vi "STED Control V7.vi"(7 "Calling VI Ref":refnum<vi>) -> ()   [LabVIEW 2016]
uses:
  FPGA-7842R-Reference.ctl
  Scan Parameters.ctl
  Manual Controls V2.ctl
  Laser Controls.ctl
  <vilib>/vision/Image Controls.llb/IMAQ Image.ctl
  <vilib>/Utility/miscctls.llb/LVPointTypeDef.ctl
  Type Defs/Image Acquisition Parameters.ctl
  Detectors.ctl
  Focus Control.ctl
panel:
  in  "File Name":string
  in  "Focus Control":T1
  in  "Detectors":T2
  in  "Laser Controls":T3 {"405 Power (0-5V)" min=0.0 max=5.0}
  in  "Save Path":path
  in  "Capture":bool
  in  "Image Acquisition Parameters":T4={"Scan Type"=enum."Beam Scanning", "Scan Mode"=enum."XY", "Fast Axis Frequency (Hz)"=16110.0, "Image Format"=256, "Line Accumulations"=100, "Frames Per Capture"=1, "Frames Accumulations"=1, "Image Dimension (um)"=[15.0, 15.0], "Number of Z Steps"=1, "Z Steps Size (um)"=1.0, "Pixel Size (nm)"=[58.59375, 58.59375]} {"Z Steps Size (um)" min=0.0; "Number of Z Steps" min=1; "Frames Accumulations" min=1; "Frames Per Capture" min=1; "Line Accumulations" min=1; "Image Format" items=["64 x 64"=64, "128 x 128"=128, "256 x 256"=256, "512 x 512"=512, "1024 x 1024"=1024, "2048 x 2048"=2048]}
  in  "Live":bool
  in  "Quit":bool
  # "Copyright (C) 2020 Edward S Allgeyer\n\nRedistribution and use in source and binary forms, with or without\nmodification, are permitted provided that the following conditions\nare met:\n\n1. Redistributions of source code must retain the above copyright\n   notice, this list of conditions and the following disclaimer.\n\n2. Redistributions in binary form must reproduce the above copyright\n   notice, this list of conditions and the following disclaimer in\n   the documentation and/or other materials provided with the\n   distribution.\n\n3. Neither the name of the copyright holder nor the names of its\n   contributors may be used to endorse or promote products derived\n   from this software without specific prior written permission.\n\nTHIS SOFTWARE IS PROVIDED BY THE COPYRIGHT HOLDERS AND CONTRIBUTORS\n\"AS IS\" AND ANY EXPRESS OR IMPLIED WARRANTIES, INCLUDING, BUT NOT\nLIMITED TO, THE IMPLIED WARRANTIES OF MERCHANTABILITY AND FITNESS\nFOR A PARTICULAR PURPOSE ARE DISCLAIMED. IN NO EVENT SHALL THE\nCOPYRIGHT HOLDER OR CONTRIBUTORS BE LIABLE FOR ANY DIRECT, INDIRECT,\nINCIDENTAL, SPECIAL, EXEMPLARY, OR CONSEQUENTIAL DAMAGES (INCLUDING,\nBUT NOT LIMITED TO, PROCUREMENT OF SUBSTITUTE GOODS OR SERVICES;\nLOSS OF USE, DATA, OR PROFITS; OR BUSINESS INTERRUPTION) HOWEVER\nCAUSED AND ON ANY THEORY OF LIABILITY, WHETHER IN CONTRACT, STRICT\nLIABILITY, OR TORT (INCLUDING NEGLIGENCE OR OTHERWISE) ARISING IN\nANY WAY OUT OF THE USE OF THIS SOFTWARE, EVEN IF ADVISED OF THE\nPOSSIBILITY OF SUCH DAMAGE."
  # "XY"
  # "Z"
  # "Length"
  # "Height"
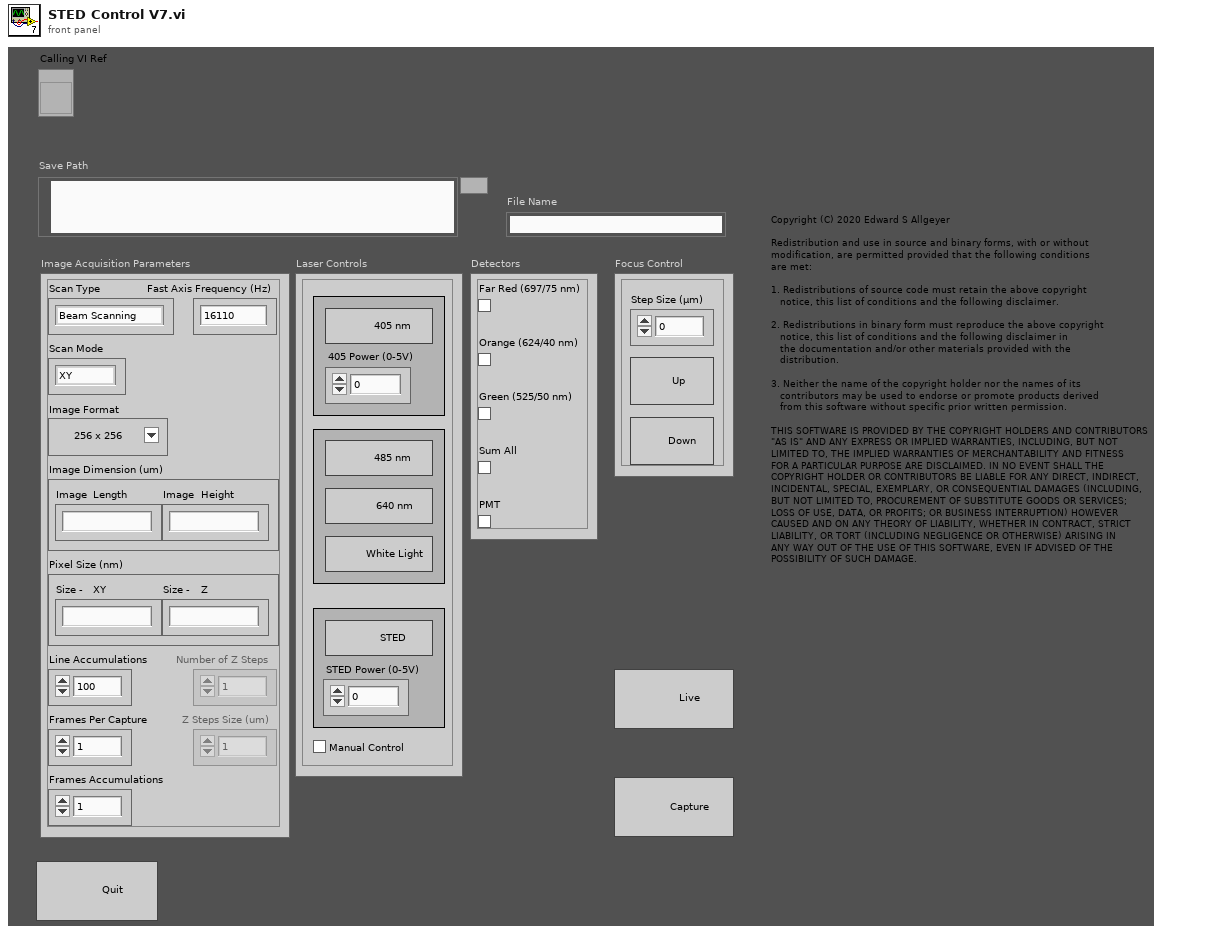
[diagram p1: front panel]
types:
  T1 = typedef "Focus Control.ctl" = cluster{"ZoomUp":bool, "ZoomDown":bool, "SetZoom":bool, "Step Size (µm)":dbl}
  T2 = typedef "Detectors.ctl" = cluster{"PMT":bool, "Far Red (697/75 nm)":bool, "Orange (624/40 nm)":bool, "Green (525/50 nm)":bool, "Sum All":bool}
  T3 = typedef "Laser Controls.ctl" = cluster{"STED Power (0-5V)":dbl, "STED":bool, "640 nm":bool, "485 nm":bool, "Manual Control":bool, "White Light":bool, "405 nm":bool, "405 Power (0-5V)":dbl}
  T4 = typedef "Image Acquisition Parameters.ctl" = cluster{"Scan Type":enum16{"Sample Scanning", "Beam Scanning"}, "Scan Mode":enum16{"XY", "XZ", "YZ", "XYZ"}, "Fast Axis Frequency (Hz)":dbl, "Image Format":u16, "Line Accumulations":u16, "Frames Per Capture":u16, "Frames Accumulations":u16, "Image Dimension (um)":dbl[], "Number of Z Steps":u8, "Z Steps Size (um)":dbl, "Pixel Size (nm)":dbl[]}
  T5 = enum8{"Enabled", "Disabled", "Disabled and Grayed Out"}
  T6 = enum16{"Always On", "Always Off", "Off While Running"}
  T7 = typedef "LVPointTypeDef.ctl" = cluster{"Horizontal":i16, "Vertical":i16}
  T8 = typedef "Manual Controls V2.ctl" = cluster{"Galvo 1 Position (I16)":i16, "Galvo 2 Position (I16)":i16, "X Axis Voltage (I16)":i16, "Y Axis Voltage (I16)":i16, "Z Axis Voltage (I16)":i16, "Res Mirror Amp (I16)":i16, "Res Mirror Mute":bool}
  T9 = typedef "Scan Parameters.ctl" = cluster{"Fast_Ax_Amp_V":dbl, "Fast_Ax_Off_V":dbl, "Slow_Ax_Amp_V":dbl, "Slow_Ax_Off_V ":dbl, "Slow_Ax_Max_V_VperS":dbl, "Slow_Ax1_Del25ns":i32, "Slow_Ax2_Del25ns":i32, "Stage_X_Off_V":dbl, "Stage_Y_Off_V":dbl, "Stage_Z_Off_V":dbl, "Galvo1_Off_V":dbl, "Galvo2_Off_V":dbl, "Last_Scan_Mode":enum16{"XY", "XZ", "YZ", "XYZ"}, "Current_Scan_Mode":enum16{"XY", "XZ", "YZ", "XYZ"}, "Fly_Back_Lines":u16, "Linear_Ramp_End":u32, "Z_Step_I16":i16, "Z_Start_I16":i16, "Laser_States _U32":u32, "590_Voltage_I16":i16, "775_AOM_Volt_I16":i16, "Blanking OFF":bool, "Unused_Axis_I16":i16}
  T10 = typedef "FPGA-7842R-Reference.ctl" = enum16{"Stage Control", "Laser Control", "Unused Axis I16", "Exit", "Set Res Mirror", "Set Galvo", "Default", "Close FPGA", "Stop Waveforms", "Start Waveforms", "Initialize"}
  T11 = typedef "LVRectTypeDef.ctl" = cluster{"Left":i16, "Top":i16, "Right":i16, "Bottom":i16}
  T12 = typedef "LVBoundsTypeDef.ctl" = cluster{"Width":u32, "Height":u32}
  T13 = cluster{"Scan Type":bool, "Scan Mode":bool, "Fast Axis Frequency (Hz)":bool, "Image Format":bool, "Line Accumulations":bool, "Frames Per Capture":bool, "Frames Accumulations":bool, "Image Dimension (um)":bool[], "Number of Z Steps":bool, "Z Steps Size (um)":bool, "Pixel Size (nm)":bool[]}
  T14 = typedef "Scanning Conversions.ctl" = cluster{"Stage X Axis (Volts/um)":dbl, "Stage Y Axis (Volts/um)":dbl, "Stage Z Axis (Volts/um)":dbl}
  T15 = typedef "IMAQ Image.ctl" = refnum<image>
  T16 = typedef "Waveform Data.ctl" = cluster{"Waveform Scan Parameters":cluster{"Scanning Mode":u8, "Fast Axis WF Length (Elements)":i32, "Fast Axis Sample Period (Ticks)":u32, "Slow Axis 1 WF Length (Elements)":i32, "Slow Axis 1 Sample Period (Ticks)":u32, "Slow Axis 1 Delay (25 ns) Steps":i32, "Slow Axis 2 WFLength (Elements)":i32, "Slow Axis 2 Sample Period (Ticks)":u32, "Slow Axis 2 Delay (25 ns) Steps":i32}, "Fast Axis Waveform":dbl[], "Slow Axis 1 Waveform":dbl[], "Slow Axis 2 Waveform":dbl[]}
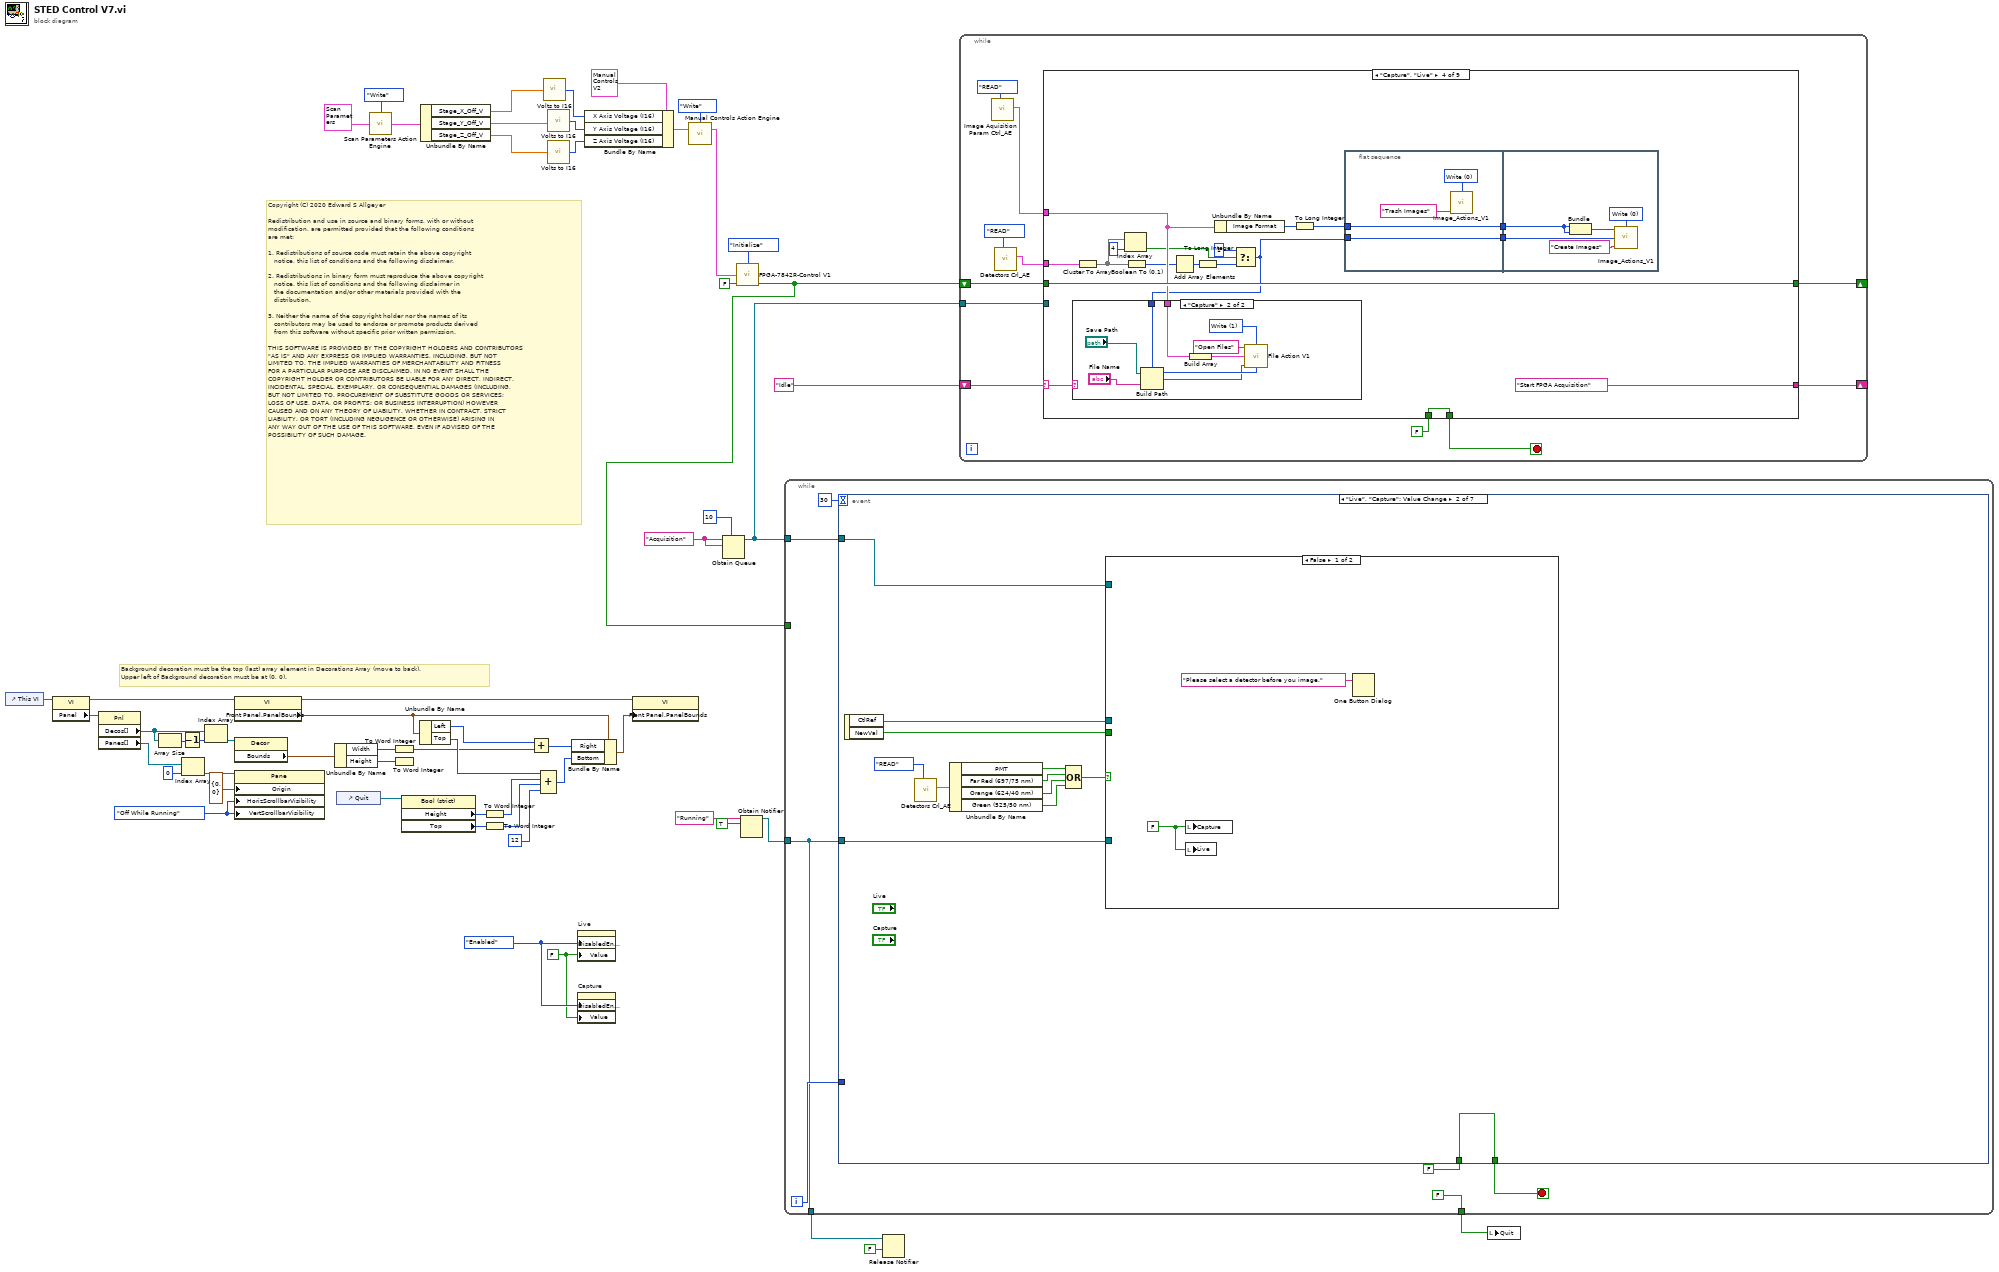
[diagram p0: block diagram]
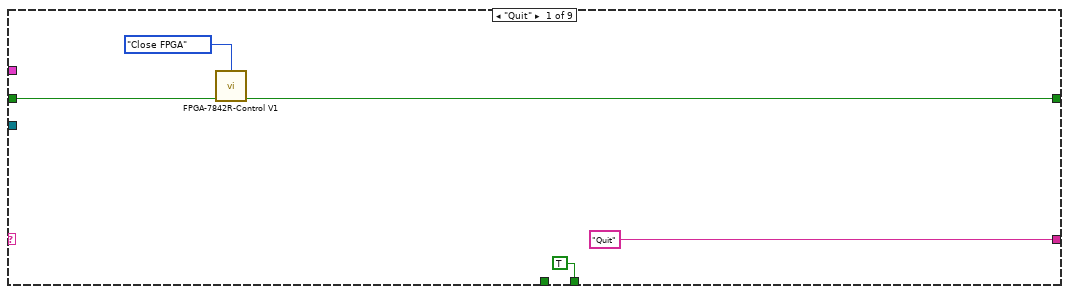
[diagram p2: hidden frame]
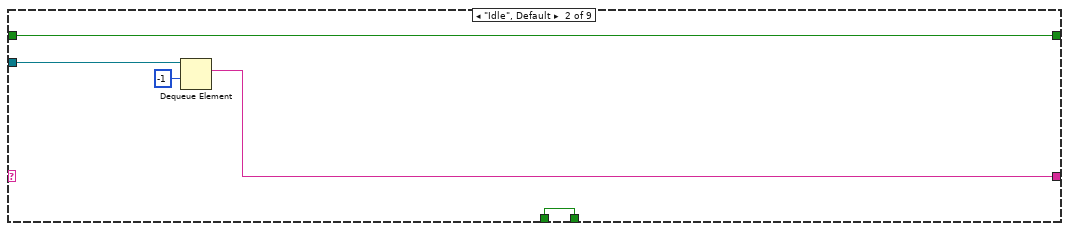
[diagram p3: hidden frame]
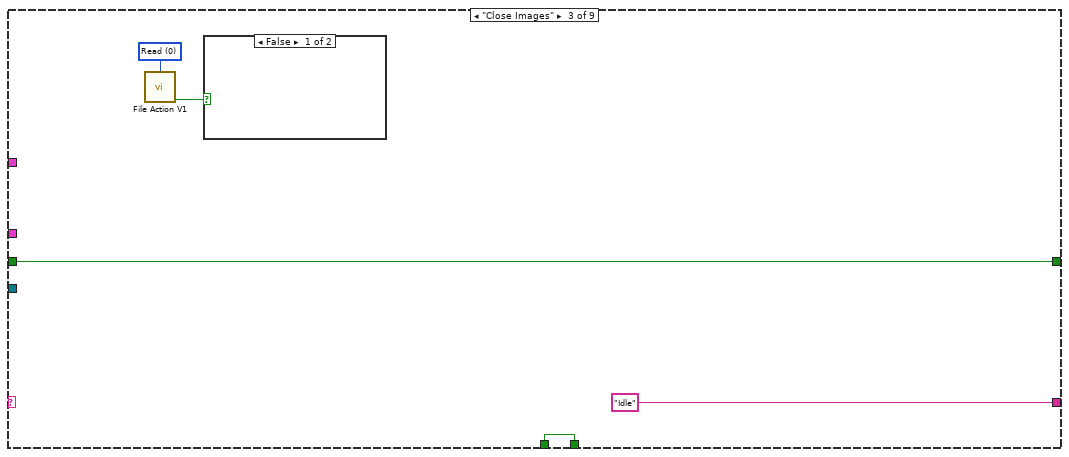
[diagram p4: hidden frame]
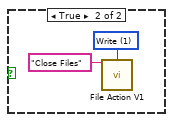
[diagram p5: hidden frame]
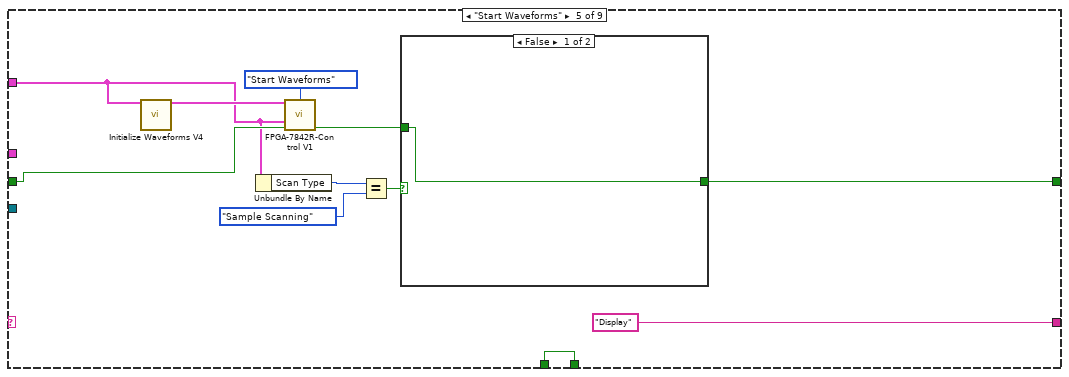
[diagram p7: hidden frame]
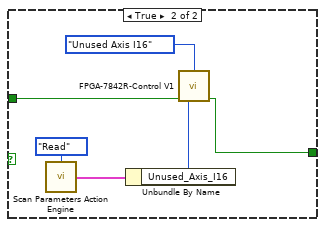
[diagram p8: hidden frame]
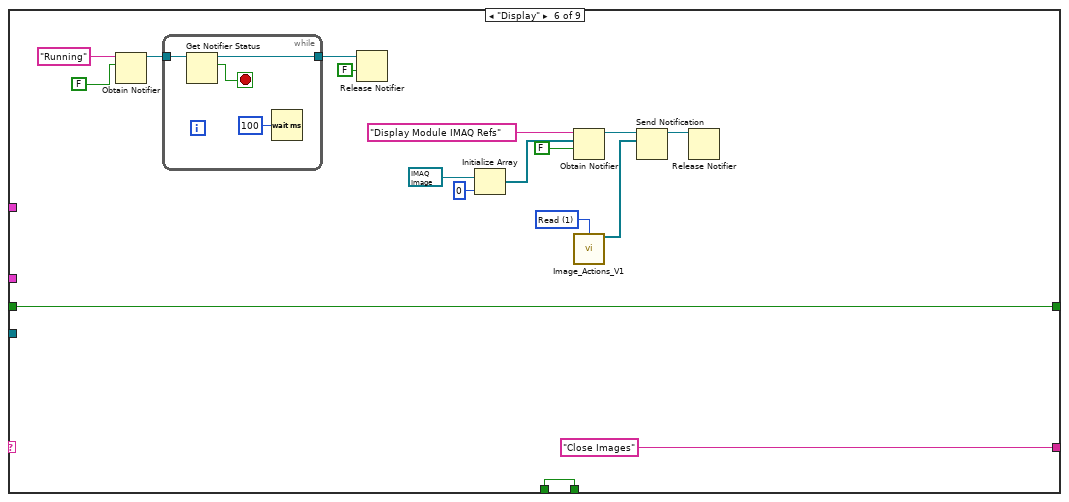
[diagram p9: hidden frame]
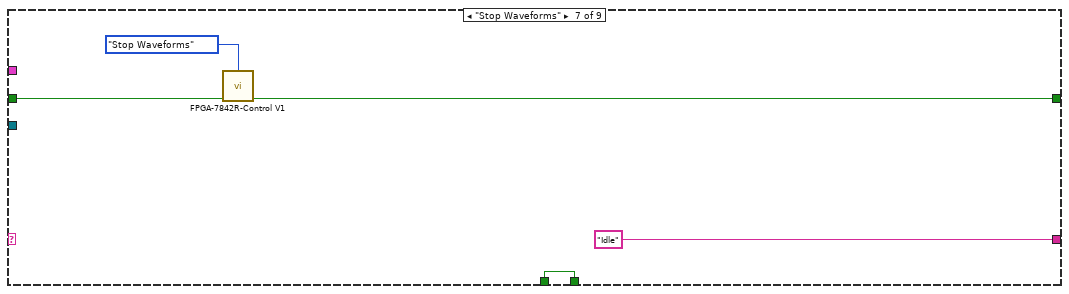
[diagram p10: hidden frame]
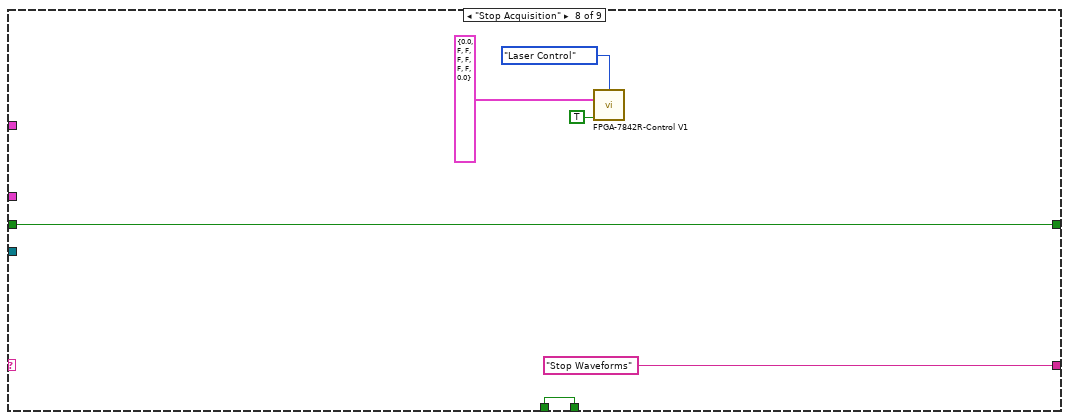
[diagram p11: hidden frame]
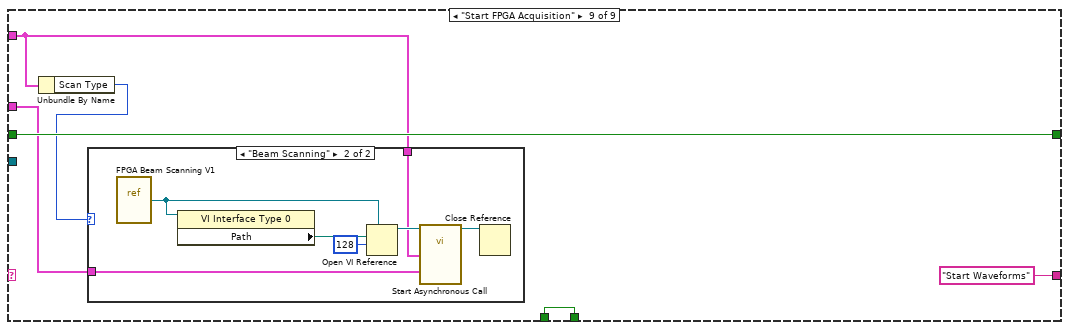
[diagram p12: hidden frame]
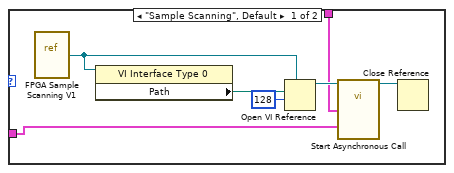
[diagram p13: hidden frame]
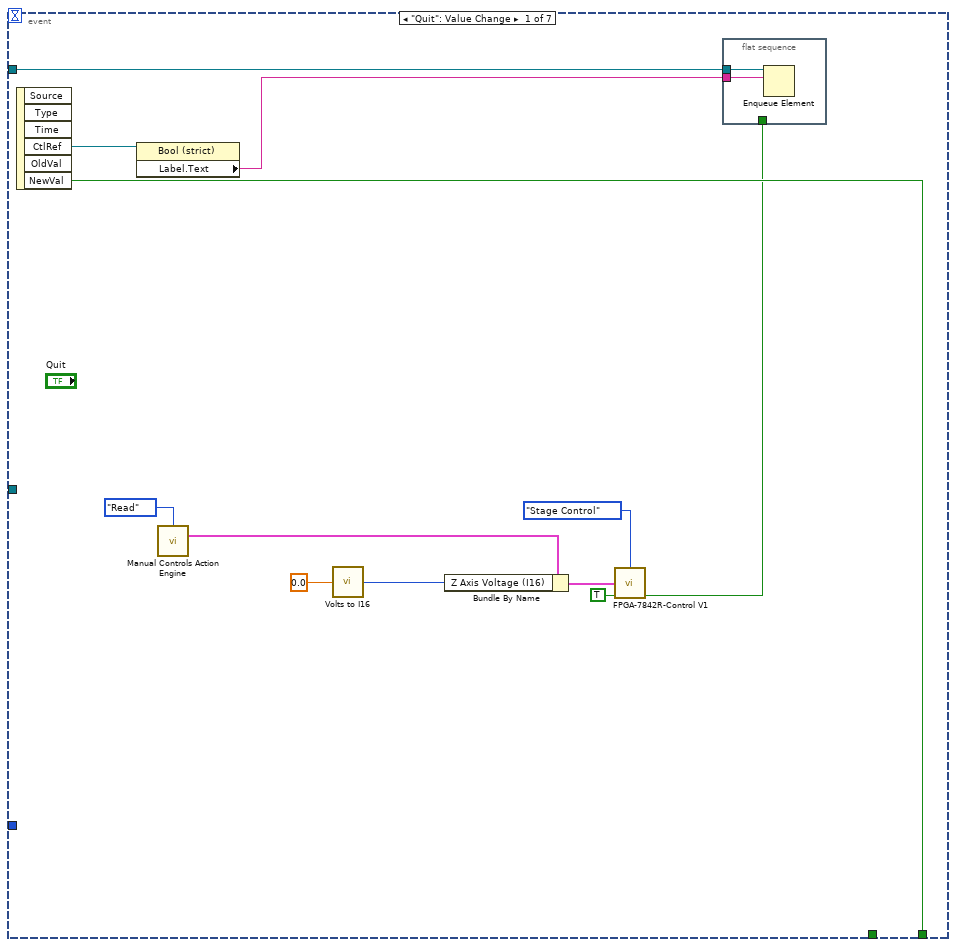
[diagram p14: hidden frame]
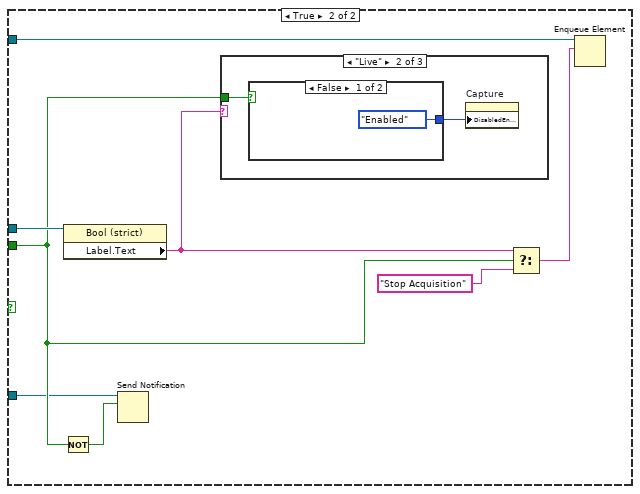
[diagram p15: hidden frame]
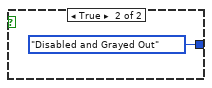
[diagram p17: hidden frame]
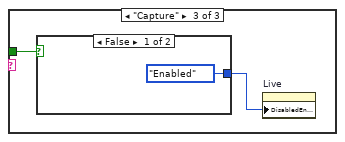
[diagram p18: hidden frame]
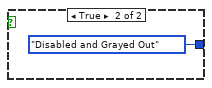
[diagram p19: hidden frame]
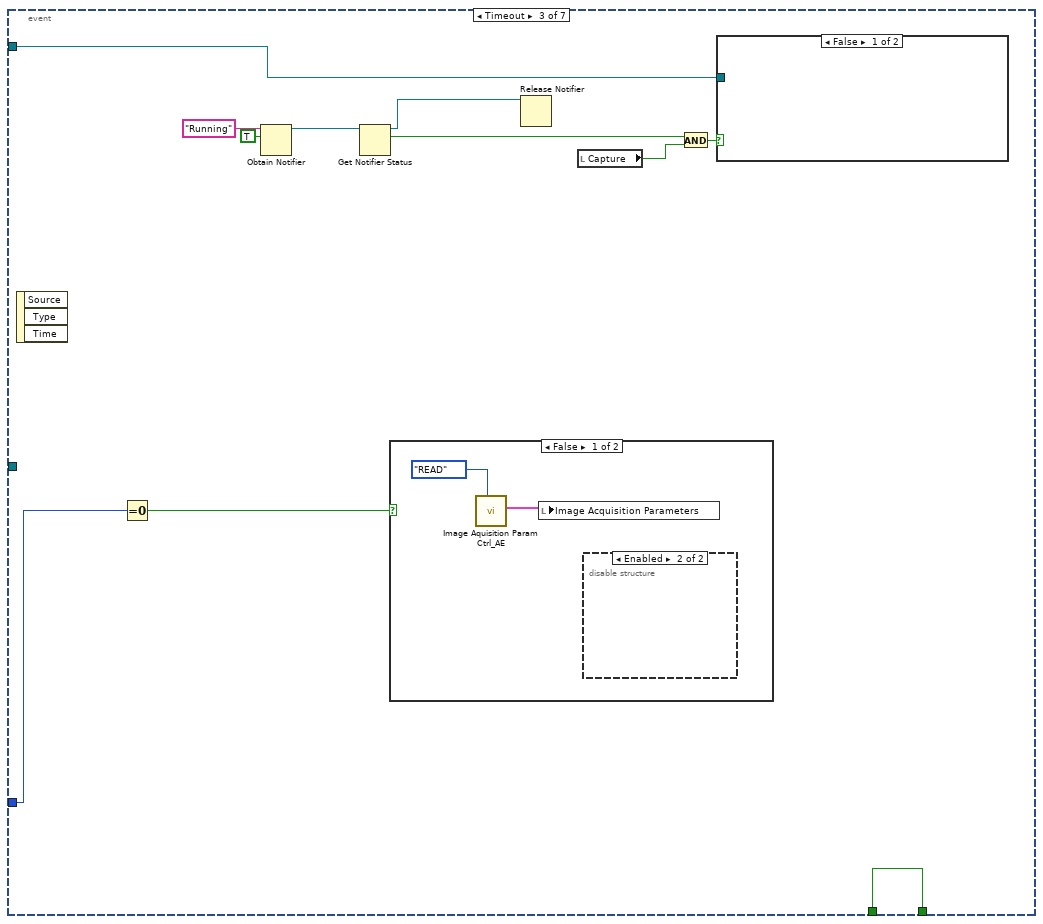
[diagram p20: hidden frame]
diagram:
  w1 = FALSE ("Live")
  w2 = T5."Enabled" ("Disabled")
  w15 = T6."Off While Running" ("Vertical Scrollbar Visibility")
  w56 = "Acquisition" ("name (unnamed)")
  # "Copyright (C) 2020 Edward S Allgeyer\n\nRedistribution and use in source and binary forms, with or without\nmodification, are permitted provided that the following conditions\nare met:\n\n1. Redistributions of source code must retain the above copyright\n   notice, this list of conditions and the following disclaimer.\n\n2. Redistributions in binary form must reproduce the above copyright\n   notice, this list of conditions and the following disclaimer in\n   the documentation and/or other materials provided with the\n   distribution.\n\n3. Neither the name of the copyright holder nor the names of its\n   contributors may be used to endorse or promote products derived\n   from this software without specific prior written permission.\n\nTHIS SOFTWARE IS PROVIDED BY THE COPYRIGHT HOLDERS AND CONTRIBUTORS\n\"AS IS\" AND ANY EXPRESS OR IMPLIED WARRANTIES, INCLUDING, BUT NOT\nLIMITED TO, THE IMPLIED WARRANTIES OF MERCHANTABILITY AND FITNESS\nFOR A PARTICULAR PURPOSE ARE DISCLAIMED. IN NO EVENT SHALL THE\nCOPYRIGHT HOLDER OR CONTRIBUTORS BE LIABLE FOR ANY DIRECT, INDIRECT,\nINCIDENTAL, SPECIAL, EXEMPLARY, OR CONSEQUENTIAL DAMAGES (INCLUDING,\nBUT NOT LIMITED TO, PROCUREMENT OF SUBSTITUTE GOODS OR SERVICES;\nLOSS OF USE, DATA, OR PROFITS; OR BUSINESS INTERRUPTION) HOWEVER\nCAUSED AND ON ANY THEORY OF LIABILITY, WHETHER IN CONTRACT, STRICT\nLIABILITY, OR TORT (INCLUDING NEGLIGENCE OR OTHERWISE) ARISING IN\nANY WAY OUT OF THE USE OF THIS SOFTWARE, EVEN IF ADVISED OF THE\nPOSSIBILITY OF SUCH DAMAGE."
  # "Background decoration must be the top (last) array element in Decorations Array (move to back).\nUpper left of Background decoration must be at (0, 0)."
  n1 = control-ref of="This VI"() -> (w7:refnum<vi>)
  n2 = property class="VI"(reference=w7) -> (reference out=w16:refnum<vi>, "Panel"=w8:refnum<vi>)  [unwired: 1 in, 1 out]
  n3 = property class="Pnl"(reference=w8) -> ("Decos[]"=w6:refnum<vi>[], "Panes[]"=w12:refnum<vi>[])  [unwired: 1 in, 2 out]
  n4 = Array Size(array=w6) -> (size(s)=w4:i32)
  n5 = Decrement(x=w4) -> (x-1=w5:i32)
  n6 = Index Array(array=w12, index=0) -> (element=w11:refnum<vi>)
  n7 = Index Array(array=w6, index=w5) -> (element=w14:refnum<vi>)
  n8 = property class="VI"(reference=w16) -> (reference out=w18:refnum<vi>, "Front Panel.PanelBounds"=w19:T11)  [unwired: 1 in, 1 out]
  n9 = property class="Decor"(reference=w14) -> ("Bounds"=w17:T12)  [unwired: 1 in, 2 out]
  n10 = property class="Pane"(reference=w11, "Origin"=T7 {"Horizontal"=0, "Vertical"=0}, "HorizScrollbarVisibility"=w15, "VertScrollbarVisibility"=w15) -> ()  [unwired: 1 in, 2 out]
  n11 = Unbundle By Name(w17) -> ("Width"=w22:u32, "Height"=w25:u32)
  n12 = control-ref of="Quit"() -> (w9:refnum<vi>)
  n13 = call "Scan Parameters Action Engine.vi"("Action"=enum16{"Read", "Write"}."Write", "Scan Parameters IN"=T9 {"Fast_Ax_Amp_V"=0.0, "Fast_Ax_Off_V"=0.0, "Slow_Ax_Amp_V"=0.0, "Slow_Ax_Off_V "=0.0, "Slow_Ax_Max_V_VperS"=0.0, "Slow_Ax1_Del25ns"=0, "Slow_Ax2_Del25ns"=0, "Stage_X_Off_V"=5.0, "Stage_Y_Off_V"=5.0, "Stage_Z_Off_V"=5.0, "Galvo1_Off_V"=0.0, "Galvo2_Off_V"=0.0, "Last_Scan_Mode"=enum."XY", "Current_Scan_Mode"=enum."XY", "Fly_Back_Lines"=0, "Linear_Ramp_End"=0, "Z_Step_I16"=0, "Z_Start_I16"=0, "Laser_States _U32"=0, "590_Voltage_I16"=0, "775_AOM_Volt_I16"=0, "Blanking OFF"=FALSE, "Unused_Axis_I16"=16384}) -> ("Scan Parameters OUT"=w45:T9)  [unwired: 13 in]
  n14 = To Word Integer(number=w22) -> (16bit integer=w24:i16)
  n15 = To Word Integer(number=w25) -> ()  [unwired: 1 out]
  n16 = property class="Bool (strict)"(reference=w9) -> ("Height"=w27:u32, "Top"=w28:i32)  [unwired: 1 in, 2 out]
  n17 = Unbundle By Name(w19) -> ("Left"=w21:i16, "Top"=w32:i16)
  n18 = Unbundle By Name(w45) -> ("Stage_X_Off_V"=w41:dbl, "Stage_Y_Off_V"=w40:dbl, "Stage_Z_Off_V"=w39:dbl)
  n19 = To Word Integer(number=w27) -> (16bit integer=w30:i16)
  n20 = To Word Integer(number=w28) -> (16bit integer=w31:i16)
  n21 = Add(x=w21, y=w24) -> (x+y=w23:i16)
  n22 = Compound Arithmetic op=ADD(w32, w30, w31, i16 12 ("y")) -> (w26:i16)
  n23 = call "Volts to I16.vi"("Voltage (V)"=w41) -> ("I16"=w42:i16)  [unwired: 13 in, 1 out]
  n24 = call "Volts to I16.vi"("Voltage (V)"=w40) -> ("I16"=w43:i16)  [unwired: 13 in, 1 out]
  n25 = call "Volts to I16.vi"("Voltage (V)"=w39) -> ("I16"=w44:i16)  [unwired: 13 in, 1 out]
  n26 = Bundle By Name(cluster=w19, "Right"=w23, "Bottom"=w26) -> (w20:T11)
  n27 = property on="Live" class="Bool (strict)"("DisabledEnum"=w2, "Value"=w1) -> ()  [unwired: 2 in, 2 out]
  n28 = property on="Capture" class="Bool (strict)"("DisabledEnum"=w2, "Value"=w1) -> ()  [unwired: 2 in, 2 out]
  n29 = Bundle By Name(cluster=T8 {"Galvo 1 Position (I16)"=-280, "Galvo 2 Position (I16)"=0, "X Axis Voltage (I16)"=16384, "Y Axis Voltage (I16)"=16384, "Z Axis Voltage (I16)"=16384, "Res Mirror Amp (I16)"=0, "Res Mirror Mute"=FALSE} ("Manual Controls"), "X Axis Voltage (I16)"=w42, "Y Axis Voltage (I16)"=w43, "Z Axis Voltage (I16)"=w44) -> (w46:T8)
  n30 = property class="VI"(reference=w18, "Front Panel.PanelBounds"=w20) -> ()  [unwired: 1 in, 2 out]
  n31 = call "Manual Controls Action Engine.vi"("Action"=enum16{"Read", "Write"}."Write", "Manual Controls In"=w46) -> ("Manual Controls Out"=w48:T8)  [unwired: 13 in]
  n32 = Obtain Queue(max queue size (-1, unlimited)=10, name (unnamed)=w56, element data type=w56) -> (queue out=w54:refnum<queue>)  [unwired: 2 in, 2 out]
  n33 = call "FPGA-7842R-Control V1.vi"("Action"=FPGA-7842R-Reference."Initialize", "Manual Controls"=w48, "Initialize"=FALSE) -> ("Initalized"=w33:bool)  [unwired: 12 in]
  n34 = Obtain Notifier(name (unnamed)="Running", notification data type=TRUE) -> (notifier out=w36:refnum<notifier>)  [unwired: 2 in, 2 out]
  n35 = while {
    tunnel: w54 -> [w62]
    tunnel: w36 -> [w59]
    tunnel: [w59] -> w34
    tunnel: w33 -> [_]
    tunnel: [FALSE] -> w3
    i -> [w60]
    stop <- w64 stop-if-true
    n36 = event shown="[1] \"Live\", \"Capture\": Value Change" {
      selector: _ -> [_ _ _ _ _ _ _]
      dyn-events: _ -> [_ _ _ _ _ _ _]
      timeout: 30 -> [_ _ _ _ _ _ _]
      tunnel: [w76 w90 w119 w138 w163 w199 w235] -> w64
      tunnel: FALSE -> [_ w90 w119 w138 w163 w199 w235]
      tunnel: w62 -> [w75 w89 w113 _ _ _ _]
      tunnel: w60 -> [_ _ w111 _ _ _ _]
      tunnel: w59 -> [_ w86 _ _ _ _ _]
      event "Quit": Value Change {
        n37 = event-data() -> ("CtlRef"=w74:refnum<vi>, "NewVal"=w76:bool)  [unwired: 1 in, 4 out]
        n38 = property class="Bool (strict)"(reference=w74) -> ("Label.Text"=w73:string)  [unwired: 1 in, 2 out]
        n39 = call "Manual Controls Action Engine.vi"("Action"=enum16{"Read", "Write"}."Read") -> ("Manual Controls Out"=w72:T8)  [unwired: 14 in]
        n40 = call "Volts to I16.vi"("Voltage (V)"=0.0) -> ("I16"=w65:i16)  [unwired: 13 in, 1 out]
        n41 = Bundle By Name(cluster=w72, "Z Axis Voltage (I16)"=w65) -> (w70:T8)
        n42 = call "FPGA-7842R-Control V1.vi"("Action"=FPGA-7842R-Reference."Stage Control", "Manual Controls"=w70, "Initialize"=TRUE) -> ("Initalized"=w66:bool)  [unwired: 12 in]
        n43 = flat-sequence {
          tunnel: w75 -> [w78]
          tunnel: w73 -> [w77]
          tunnel: w66 -> [_]
          frame #0 {
            n44 = Enqueue Element(queue=w78, element=w77) -> ()  [unwired: 2 in, 3 out]
          }
        }
      }
      event "Live", "Capture": Value Change {
        n45 = event-data() -> ("CtlRef"=w88:refnum<vi>, "NewVal"=w87:bool)  [unwired: 1 in]
        n46 = call "Detectors Crl_AE.vi"("Action"=enum16{"READ", "WRITE"}."READ") -> ("Detectors Parameters Out"=w84:T2)  [unwired: 10 in]
        n47 = Unbundle By Name(w84) -> ("PMT"=w83:bool, "Far Red (697/75 nm)"=w82:bool, "Orange (624/40 nm)"=w81:bool, "Green (525/50 nm)"=w80:bool)
        n48 = Compound Arithmetic op=OR(w83, w82, w81, w80) -> (w79:bool)
        n49 = case shown="False" w79 {
          tunnel: w89 -> [_ w100]
          tunnel: w88 -> [_ w99]
          tunnel: w87 -> [_ w94]
          tunnel: w86 -> [_ w93]
          frame False {
            w92 = FALSE ("Capture")
            n50 = local write "Capture"(w92) -> ()
            n51 = local write "Live"(w92) -> ()
            n52 = One Button Dialog(message="Please select a detector before you image.") -> ()  [unwired: 1 in, 1 out]
          }
          frame True {
            n53 = Not(x=w94) -> (.not. x?=w97:bool)
            n54 = property class="Bool (strict)"(reference=w99) -> ("Label.Text"=w95:string)  [unwired: 1 in, 2 out]
            n55 = Send Notification(notification=w97, notifier=w93) -> ()  [unwired: 1 in, 2 out]
            n56 = case shown="\"Live\"" w95 {
              tunnel: w94 -> [_ w101 w106]
              frame "False", Default {
              }
              frame "Live" {
                n57 = case shown="False" w101 {
                  tunnel: [T5."Enabled" ("Disabled") T5."Disabled and Grayed Out" ("Disabled")] -> w102
                  frame False {
                  }
                  frame True {
                  }
                }
                n58 = property on="Capture" class="Bool (strict)"("DisabledEnum"=w102) -> ()  [unwired: 2 in, 2 out]
              }
              frame "Capture" {
                n59 = case shown="False" w106 {
                  tunnel: [T5."Enabled" ("Disabled") T5."Disabled and Grayed Out" ("Disabled")] -> w105
                  frame False {
                  }
                  frame True {
                  }
                }
                n60 = property on="Live" class="Bool (strict)"("DisabledEnum"=w105) -> ()  [unwired: 2 in, 2 out]
              }
            }
            n61 = Select(t=w95, s=w94, f="Stop Acquisition") -> (s? t:f=w96:string)
            n62 = Enqueue Element(queue=w100, element=w96) -> ()  [unwired: 2 in, 3 out]
          }
        }
      }
      event Timeout {
        n63 = event-data() -> ()  [unwired: 1 in, 3 out]
        n64 = Equal To 0?(x=w111) -> (x = 0?=w110:bool)
        n65 = Obtain Notifier(name (unnamed)="Running", notification data type=TRUE) -> (notifier out=w117:refnum<notifier>)  [unwired: 2 in, 2 out]
        n66 = Get Notifier Status(notifier=w117) -> (notifier out=w109:refnum<notifier>, current notification=w115:bool)  [unwired: 1 in, 3 out]
        n67 = case shown="False" w110 {
          frame False {
            n68 = call "Image Aquisition Param Ctrl_AE.vi"("Action"=enum16{"READ", "WRITE"}."READ") -> ("Image Acquisition Parameters Out"=w121:T4)  [unwired: 10 in]
            n69 = local write "Image Acquisition Parameters"(w121) -> ()
            n70 = disable-structure shown="Enabled" {
              frame Disabled {
                n71 = call "FPGA-7842R-Control V1.vi"("Action"=FPGA-7842R-Reference."Exit", "Initialize"=TRUE) -> ()  [unwired: 13 in, 1 out]
              }
              frame Enabled {
              }
            }
          }
          frame True {
            n72 = local read "Image Acquisition Parameters"() -> (w124:T4)
            n73 = call "Image Aquisition Param Ctrl_AE.vi"("Action"=enum16{"READ", "WRITE"}."WRITE", "Image Acquisition Parameters In"=w124) -> ()  [unwired: 9 in, 1 out]
          }
        }
        n74 = Release Notifier(notifier=w109) -> ()  [unwired: 2 in, 3 out]
        n75 = local read "Capture"() -> (w114:bool)
        n76 = And(x=w115, y=w114) -> (x .and. y?=w112:bool)
        n77 = case shown="False" w112 {
          tunnel: w113 -> [_ w128]
          frame False {
          }
          frame True {
            n78 = local write "Capture"(FALSE ("Capture")) -> ()
            n79 = Enqueue Element(queue=w128, element="Stop Acquisition" ("f")) -> ()  [unwired: 2 in, 3 out]
            n80 = property on="Live" class="Bool (strict)"("DisabledEnum"=T5."Enabled" ("Disabled")) -> ()  [unwired: 2 in, 2 out]
          }
        }
      }
      event Value Change {
        w150 = FALSE ("element")
        n81 = event-data() -> ()  [unwired: 1 in, 6 out]
        n82 = Unbundle By Name("Laser Controls") -> ("405 nm"=w132:bool, "STED"=w155:bool, "640 nm"=w153:bool, "White Light"=w133:bool, "485 nm"=w154:bool, "STED Power (0-5V)"=w147:dbl, "405 Power (0-5V)"=w130:dbl, "Manual Control"=w131:bool)
        n83 = call "LASERs_ Crl_AE.vi"("Action"=enum16{"READ", "WRITE"}."WRITE", "Laser Parameters In"="Laser Controls") -> ()  [unwired: 9 in, 1 out]
        n84 = Build Array(w155, w153, w132, w154, w133, w150, w150, w150) -> (w152:bool[])
        n85 = local read "Live"() -> (w137:bool)
        n86 = Boolean Array To Number(Boolean array=w152) -> (number=w151:u32)
        n87 = To Unsigned Byte Integer(number=w151) -> (unsigned 8bit integer=w149:u8)
        n88 = Or(x=w137, y=w131) -> (x .or. y?=w136:bool)
        n89 = In Range and Coerce(upper limit=5.0, x=w130, lower limit=0.0) -> (coerced(x)=w142:dbl)  [unwired: 1 out]
        n90 = In Range and Coerce(upper limit=5.0, x=w147, lower limit=0.0) -> (coerced(x)=w141:dbl)  [unwired: 1 out]
        n91 = call "U8_To_U32.vi"("U8 IN"=w149) -> ("U32 OUT"=w148:u32)  [unwired: 13 in, 1 out]
        n92 = call "Volts to I16.vi"("Voltage (V)"=w142) -> ("I16"=w140:i16)  [unwired: 13 in, 1 out]
        n93 = call "Volts to I16.vi"("Voltage (V)"=w141) -> ("I16"=w139:i16)  [unwired: 13 in, 1 out]
        n94 = case shown="True" w136 {
          tunnel: "Laser Controls" -> [_ w161]
          frame False {
          }
          frame True {
            n95 = call "FPGA-7842R-Control V1.vi"("Action"=FPGA-7842R-Reference."Laser Control", "Laser Controls"=w161, "Initialize"=TRUE) -> ()  [unwired: 12 in, 1 out]
          }
        }
        n96 = call "Scan Parameters Action Engine.vi"("Action"=enum16{"Read", "Write"}."Read") -> ("Scan Parameters OUT"=w158:T9)  [unwired: 14 in]
        n97 = Bundle By Name(cluster=w158, "Laser_States _U32"=w148, "590_Voltage_I16"=w140, "775_AOM_Volt_I16"=w139) -> (w156:T9)
        n98 = call "Scan Parameters Action Engine.vi"("Action"=enum16{"Read", "Write"}."Write", "Scan Parameters IN"=w156) -> ()  [unwired: 13 in, 1 out]
      }
      event Value Change {
        n99 = event-data() -> ()  [unwired: 1 in, 6 out]
        n100 = call "Detectors Crl_AE.vi"("Action"=enum16{"READ", "WRITE"}."WRITE", "Detectors Parameters In"="Detectors") -> ()  [unwired: 9 in, 1 out]
      }
      event Value Change {
        n101 = event-data() -> ("OldVal"=w186:T4, "NewVal"=w180:T4)  [unwired: 1 in]
        n102 = Not Equal?(x=w186, y=w180) -> (x != y?=w185:T13)
        n103 = Unbundle By Name(w185) -> ("Image Dimension (um)"=w167:bool[], "Image Format"=w175:bool, "Pixel Size (nm)"=w166:bool[])  [unwired: 1 out]
        n104 = Or Array Elements(Boolean array=w166) -> (logical OR=w179:bool)
        n105 = case shown="True" w179 {
          tunnel: w180 -> [w200 w208]
          tunnel: [w200 w206] -> w178
          tunnel: w166 -> [_ w204]
          frame False {
          }
          frame True {
            n106 = Unbundle By Name(w208) -> ("Pixel Size (nm)"=w203:dbl[], "Image Format"=w212:u16)
            n107 = for {
              tunnel: w204 -> [w213] mode=indexing
              tunnel: w203 -> [w214] mode=indexing
              tunnel: [w214] -> w205
              stop <- w213 stop-if-true
            }
            n108 = Array Size(array=w203) -> (size(s)=w202:i32)
            n109 = To Double Precision Float(number=w212) -> (double precision float=w210:dbl)
            n110 = Initialize Array(w205, w202) -> (w201:dbl[])
            n111 = Multiply(x=w201, y=w210) -> (x*y=w211:dbl[])
            n112 = Multiply(x=w211, y=0.001) -> (x*y=w207:dbl[])
            n113 = Bundle By Name(cluster=w208, "Pixel Size (nm)"=w201, "Image Dimension (um)"=w207) -> (w206:T4)
          }
        }
        n114 = Or Array Elements(Boolean array=w167) -> (logical OR=w177:bool)
        n115 = Or(x=w177, y=w175) -> (x .or. y?=w176:bool)
        n116 = case shown="True" w176 {
          tunnel: w178 -> [w215 w223]
          tunnel: [w215 w221] -> w170
          tunnel: w167 -> [_ w220]
          frame False {
          }
          frame True {
            n117 = Unbundle By Name(w223) -> ("Image Dimension (um)"=w217:dbl[], "Image Format"=w227:u16)
            n118 = for {
              tunnel: w220 -> [w228] mode=indexing
              tunnel: w217 -> [w229] mode=indexing
              tunnel: [w229] -> w219
              stop <- w228 stop-if-true
            }
            n119 = Array Size(array=w217) -> (size(s)=w216:i32)
            n120 = To Double Precision Float(number=w227) -> (double precision float=w225:dbl)
            n121 = Initialize Array(w219, w216) -> (w218:dbl[])
            n122 = Divide(x=w218, y=w225) -> (x/y=w226:dbl[])
            n123 = Multiply(x=w226, y=1000.0) -> (x*y=w222:dbl[])
            n124 = Bundle By Name(cluster=w223, "Image Dimension (um)"=w218, "Pixel Size (nm)"=w222) -> (w221:T4)
          }
        }
        n125 = Unbundle By Name(w170) -> ("Image Dimension (um)"=w187:dbl[], "Scan Type"=w192:enum16{"Sample Scanning", "Beam Scanning"})
        n126 = Equal?(x=w192, y=enum16{"Sample Scanning", "Beam Scanning"}."Beam Scanning") -> (x = y?=w171:bool)
        n127 = Index Array(array=w187, index=0) -> (element=w194:dbl)
        n128 = call "Res Mirror um to Volts.vi"("Image Size (um)"=w194) -> ("Voltage (V)"=w195:dbl)
        n129 = Select(t=16110.0, s=w171, f=100.0) -> (s? t:f=w172:dbl)
        n130 = In Range and Coerce(upper limit=5.0, x=w195, lower limit=0.0) -> (coerced(x)=w196:dbl)  [unwired: 1 out]
        n131 = Bundle By Name(cluster=w170, "Fast Axis Frequency (Hz)"=w172) -> (w169:T4)
        n132 = call "Volts to I16.vi"("Voltage (V)"=w196) -> ("I16"=w191:i16)  [unwired: 13 in, 1 out]
        n133 = call "Manual Controls Action Engine.vi"("Action"=enum16{"Read", "Write"}."Read") -> ("Manual Controls Out"=w183:T8)  [unwired: 14 in]
        n134 = Bundle By Name(cluster=w183, "Res Mirror Amp (I16)"=w191, "Res Mirror Mute"=w171) -> (w181:T8)
        n135 = call "Image Aquisition Param Ctrl_AE.vi"("Action"=enum16{"READ", "WRITE"}."WRITE", "Image Acquisition Parameters In"=w169) -> ()  [unwired: 9 in, 1 out]
        n136 = call "FPGA-7842R-Control V1.vi"("Action"=FPGA-7842R-Reference."Set Res Mirror", "Manual Controls"=w181, "Initialize"=TRUE) -> ()  [unwired: 12 in, 1 out]
        n137 = call "Manual Controls Action Engine.vi"("Action"=enum16{"Read", "Write"}."Write", "Manual Controls In"=w181) -> ()  [unwired: 13 in, 1 out]
      }
      event Value Change {
        n138 = event-data() -> ("CtlRef"=w234:refnum<vi>)  [unwired: 1 in, 2 out]
        n139 = property class="Ctl"(reference=w234) -> ("Label.Text"=w233:string)  [unwired: 1 in, 2 out]
        n140 = call "Image Aquisition Param Ctrl_AE.vi"("Action"=enum16{"READ", "WRITE"}."READ") -> ("Image Acquisition Parameters Out"=w231:T4)  [unwired: 10 in]
        n141 = case shown="\"ZoomDown\", \"ZoomUp\", Default" w233 {
          selector: w233 -> [w242]
          tunnel: w231 -> [w256]
          tunnel: "Focus Control" -> [w255]
          frame "ZoomDown", "ZoomUp", Default {
            n142 = Unbundle By Name(w255) -> ("Step Size (µm)"=w247:dbl)
            n143 = call "Scanning Volts to Microns.vi"() -> ("Scanning Conversions OUT"=w248:T14)
            n144 = Unbundle By Name(w256) -> ("Scan Type"=w254:enum16{"Sample Scanning", "Beam Scanning"}, "Scan Mode"=w253:enum16{"XY", "XZ", "YZ", "XYZ"})
            n145 = Unbundle By Name(w248) -> ("Stage Z Axis (Volts/um)"=w246:dbl)
            n146 = Equal?(x=w242, y="ZoomUp") -> (x = y?=w240:bool)
            n147 = Multiply(x=w246, y=w247) -> (x*y=w237:dbl)
            n148 = In Range and Coerce(upper limit=10.0, x=w237, lower limit=0.0) -> (coerced(x)=w236:dbl)  [unwired: 1 out]
            n149 = call "Volts to I16.vi"("Voltage (V)"=w236) -> ("I16"=w244:i16)  [unwired: 13 in, 1 out]
            n150 = Negate(x=w244) -> (-x=w243:i16)
            n151 = Select(t=w244, s=w240, f=w243) -> (s? t:f=w245:i16)
            n152 = call "Manual Controls Action Engine.vi"("Action"=enum16{"Read", "Write"}."Read") -> ("Manual Controls Out"=w252:T8)  [unwired: 14 in]
            n153 = case shown="\"Beam Scanning\"" w254 {
              tunnel: w253 -> [w267 w293]
              tunnel: w252 -> [w266 w292]
              tunnel: [w265 w289] -> w251
              tunnel: w245 -> [w257 w288]
              frame "Sample Scanning", Default {
                n154 = case shown="\"XZ\"" w267 {
                  tunnel: w266 -> [w272 w277 w282 w287]
                  tunnel: w257 -> [w270 w275 w280 w285]
                  tunnel: [w269 w274 w279 w284] -> w265
                  tunnel: [w268 w273 w278 w283] -> w262
                  frame "XZ" {
                    n155 = Unbundle By Name(w272) -> ("Y Axis Voltage (I16)"=w271:i16)
                    n156 = Add(x=w271, y=w270) -> (x+y=w268:i16)
                    n157 = Bundle By Name(cluster=w272, "Y Axis Voltage (I16)"=w268) -> (w269:T8)
                  }
                  frame "YZ" {
                    n158 = Unbundle By Name(w277) -> ("X Axis Voltage (I16)"=w276:i16)
                    n159 = Add(x=w276, y=w275) -> (x+y=w273:i16)
                    n160 = Bundle By Name(cluster=w277, "X Axis Voltage (I16)"=w273) -> (w274:T8)
                  }
                  frame "XYZ" {
                    n161 = Unbundle By Name(w282) -> ("Z Axis Voltage (I16)"=w281:i16)
                    n162 = Add(x=w281, y=w280) -> (x+y=w278:i16)
                    n163 = Bundle By Name(cluster=w282, "Z Axis Voltage (I16)"=w278) -> (w279:T8)
                  }
                  frame "XY" {
                    n164 = Unbundle By Name(w287) -> ("Z Axis Voltage (I16)"=w286:i16)
                    n165 = Add(x=w286, y=w285) -> (x+y=w283:i16)
                    n166 = Bundle By Name(cluster=w287, "Z Axis Voltage (I16)"=w283) -> (w284:T8)
                  }
                }
                n167 = call "FPGA-7842R-Control V1.vi"("Action"=FPGA-7842R-Reference."Unused Axis I16", "Initialize"=TRUE, "Unused Axis Offset (I16)"=w262) -> ()  [unwired: 12 in, 1 out]
                n168 = call "Scan Parameters Action Engine.vi"("Action"=enum16{"Read", "Write"}."Read") -> ("Scan Parameters OUT"=w261:T9)  [unwired: 14 in]
                n169 = Bundle By Name(cluster=w261, "Unused_Axis_I16"=w262) -> (w260:T9)
                n170 = call "Scan Parameters Action Engine.vi"("Action"=enum16{"Read", "Write"}."Write", "Scan Parameters IN"=w260) -> ()  [unwired: 13 in, 1 out]
              }
              frame "Beam Scanning" {
                n171 = case shown="\"XY\", Default" w293 {
                  tunnel: w292 -> [w298]
                  tunnel: [w297] -> w289
                  tunnel: w288 -> [w296]
                  frame "XY", Default {
                    n172 = Unbundle By Name(w298) -> ("Z Axis Voltage (I16)"=w295:i16)
                    n173 = call "CheckI16_Range.vi"("Step"=w296, "Current"=w295) -> ("In Range Value"=w294:i16)  [unwired: 9 in]
                    n174 = Bundle By Name(cluster=w298, "Z Axis Voltage (I16)"=w294) -> (w297:T8)
                  }
                }
                n175 = call "FPGA-7842R-Control V1.vi"("Action"=FPGA-7842R-Reference."Stage Control", "Manual Controls"=w289, "Initialize"=TRUE) -> ()  [unwired: 12 in, 1 out]
              }
            }
            n176 = call "Manual Controls Action Engine.vi"("Action"=enum16{"Read", "Write"}."Write", "Manual Controls In"=w251) -> ()  [unwired: 13 in, 1 out]
          }
        }
      }
    }
  }
  n177 = Release Notifier(notifier=w34, force destroy? (F)=FALSE) -> ()  [unwired: 1 in, 3 out]
  n178 = while {
    shift-right: [w308] -> _
    shift-left: "Idle" -> [w309]
    tunnel: w54 -> [w305]
    shift-right: [w303] -> _
    shift-left: w33 -> [w304]
    stop <- w307 stop-if-true
    n179 = call "Image Aquisition Param Ctrl_AE.vi"("Action"=enum16{"READ", "WRITE"}."READ") -> ("Image Acquisition Parameters Out"=w302:T4)  [unwired: 10 in]
    n180 = call "Detectors Crl_AE.vi"("Action"=enum16{"READ", "WRITE"}."READ") -> ("Detectors Parameters Out"=w300:T2)  [unwired: 10 in]
    n181 = case shown="\"Capture\", \"Live\"" w309 {
      selector: w309 -> [_ _ _ w340 _ _ _ _ _]
      tunnel: ["Quit" w316 "Idle" ("name (unnamed)") "Start FPGA Acquisition" ("name (unnamed)") "Display" ("name (unnamed)") "Close Images" ("name (unnamed)") "Idle" "Stop Waveforms" ("name (unnamed)") "Start Waveforms" ("name (unnamed)")] -> w308
      tunnel: [TRUE w318 w323 w344 w372 w396 w405 w410 w416] -> w307
      tunnel: FALSE -> [_ w318 w323 w344 w372 w396 w405 w410 w416]
      tunnel: w305 -> [_ w317 _ _ _ _ _ _ _]
      tunnel: w304 -> [w312 w315 w324 w343 w370 w394 w403 w411 w417]
      tunnel: [w311 w315 w324 w343 w366 w394 w402 w411 w417] -> w303
      tunnel: w302 -> [_ _ _ w339 w365 _ _ _ w414]
      tunnel: w300 -> [_ _ _ w338 _ _ _ _ w412]
      frame "Quit" {
        n182 = call "FPGA-7842R-Control V1.vi"("Action"=FPGA-7842R-Reference."Close FPGA", "Initialize"=w312) -> ("Initalized"=w311:bool)  [unwired: 13 in]
      }
      frame "Idle", Default {
        n183 = Dequeue Element(queue=w317, timeout in ms (-1)=-1) -> (element=w316:string)  [unwired: 1 in, 3 out]
      }
      frame "Close Images" {
        w321 = u16 0 items=["Read", "Write"] ("Mode")
        n184 = call "File Action V1.vi"("Mode"=w321) -> ("Files Open"=w320:bool)  [unwired: 12 in, 2 out]
        n185 = case shown="False" w320 {
          frame False {
          }
          frame True {
            w326 = u16 1 items=["Read", "Write"] ("Mode")
            n186 = call "File Action V1.vi"("Action"="Close Files", "Mode"=w326) -> ()  [unwired: 11 in, 3 out]
          }
        }
      }
      frame "Capture", "Live" {
        n187 = Cluster To Array(cluster=w338) -> (array=w336:bool[])
        n188 = Index Array(array=w336, index=4) -> (element=w333:bool)
        n189 = Boolean To (0,1)(Boolean=w336) -> (0, 1=w337:i16[])
        n190 = Add Array Elements(numeric array=w337) -> (sum=w334:i16)
        n191 = To Long Integer(number=w334) -> (32bit integer=w331:i32)
        n192 = Unbundle By Name(w339) -> ("Image Format"=w341:u16)
        n193 = Select(t=1, s=w333, f=w331) -> (s? t:f=w330:i32)
        n194 = case shown="\"Capture\"" w340 {
          tunnel: w339 -> [_ w359]
          tunnel: w330 -> [_ w358]
          frame Default {
          }
          frame "Capture" {
            w360 = u16 1 items=["Read", "Write"] ("Mode")
            n195 = Build Path(base path="Save Path", name or relative path="File Name") -> (appended path=w356:path)
            n196 = Build Array(w359) -> (w357:T4[])
            n197 = call "File Action V1.vi"("Action"="Open Files", "Mode"=w360, "Image Acquisition Parameters Array"=w357, "File Path IN"=w356, "Number of Channels"=w358) -> ()  [unwired: 8 in, 3 out]
          }
        }
        n198 = To Long Integer(number=w341) -> (32bit integer=w342:i32)
        n199 = flat-sequence {
          tunnel: w330 -> [w347]
          tunnel: w342 -> [w348]
          tunnel: [w348] -> w328
          tunnel: [w347] -> w327
          tunnel: w328 -> [w351]
          tunnel: w327 -> [w349]
          frame #0 {
            w345 = u16 0 items=["Write", "Read"] ("Mode")
            n200 = call "Image_Actions_V1.vi"("Mode"=w345, "Action"="Trash Images") -> ()  [unwired: 12 in, 2 out]
          }
          frame #1 {
            w352 = u16 0 items=["Write", "Read"] ("Mode")
            n201 = Bundle(w351, w351) -> (w350:cluster{i32, i32})  [unwired: 1 in]
            n202 = call "Image_Actions_V1.vi"("Image Size (Pixels)"=w350, "Mode"=w352, "Number of Channels"=w349, "Action"="Create Images") -> ()  [unwired: 10 in, 2 out]
          }
        }
      }
      frame "Start Waveforms" {
        n203 = call "Initialize Waveforms V4.vi"("Image Acquisition Parameters"=w365) -> ("Waveform Data to FPGA"=w371:T16)  [unwired: 14 in]
        n204 = Unbundle By Name(w365) -> ("Scan Type"=w364:enum16{"Sample Scanning", "Beam Scanning"})
        n205 = call "FPGA-7842R-Control V1.vi"("Waveform Data"=w371, "Action"=FPGA-7842R-Reference."Start Waveforms", "Image Acquisition Parameters"=w365, "Initialize"=w370) -> ("Initalized"=w367:bool)  [unwired: 11 in]
        n206 = Equal?(x=w364, y=enum16{"Sample Scanning", "Beam Scanning"}."Sample Scanning" ("Scan Type")) -> (x = y?=w362:bool)
        n207 = case shown="False" w362 {
          tunnel: w367 -> [w373 w378]
          tunnel: [w373 w377] -> w366
          frame False {
          }
          frame True {
            n208 = call "Scan Parameters Action Engine.vi"("Action"=enum16{"Read", "Write"}."Read") -> ("Scan Parameters OUT"=w375:T9)  [unwired: 14 in]
            n209 = Unbundle By Name(w375) -> ("Unused_Axis_I16"=w374:i16)
            n210 = call "FPGA-7842R-Control V1.vi"("Action"=FPGA-7842R-Reference."Unused Axis I16", "Initialize"=w378, "Unused Axis Offset (I16)"=w374) -> ("Initalized"=w377:bool)  [unwired: 12 in]
          }
        }
      }
      frame "Display" {
        w390 = u16 1 items=["Write", "Read"] ("Mode")
        n211 = Obtain Notifier(name (unnamed)="Running", notification data type=FALSE) -> (notifier out=w393:refnum<notifier>)  [unwired: 2 in, 2 out]
        n212 = while {
          tunnel: w393 -> [w398]
          tunnel: [w397] -> w389
          stop <- w399 stop-if-true
          n213 = Get Notifier Status(notifier=w398) -> (notifier out=w397:refnum<notifier>, current notification=w399:bool)  [unwired: 1 in, 3 out]
          n214 = Wait (ms)(milliseconds to wait=u32 100) -> ()  [unwired: 1 out]
        }
        n215 = Release Notifier(notifier=w389, force destroy? (F)=FALSE) -> ()  [unwired: 1 in, 3 out]
        n216 = Initialize Array(T15 refnum ("New Image"), 0 ("dimension size")) -> (w383:T15[])
        n217 = Obtain Notifier(name (unnamed)="Display Module IMAQ Refs", notification data type=w383, create if not found? (T)=FALSE) -> (notifier out=w382:refnum<notifier>)  [unwired: 1 in, 2 out]
        n218 = call "Image_Actions_V1.vi"("Mode"=w390) -> ("Image REFs OUT"=w381:T15[])  [unwired: 13 in, 1 out]
        n219 = Send Notification(notification=w381, notifier=w382) -> (notifier out=w380:refnum<notifier>)  [unwired: 1 in, 1 out]
        n220 = Release Notifier(notifier=w380) -> ()  [unwired: 2 in, 3 out]
      }
      frame "Stop Waveforms" {
        n221 = call "FPGA-7842R-Control V1.vi"("Action"=FPGA-7842R-Reference."Stop Waveforms", "Initialize"=w403) -> ("Initalized"=w402:bool)  [unwired: 13 in]
      }
      frame "Stop Acquisition" {
        n222 = call "FPGA-7842R-Control V1.vi"("Action"=FPGA-7842R-Reference."Laser Control", "Laser Controls"=T3 {"STED Power (0-5V)"=0.0, "STED"=FALSE, "640 nm"=FALSE, "485 nm"=FALSE, "Manual Control"=FALSE, "White Light"=FALSE, "405 nm"=FALSE, "405 Power (0-5V)"=0.0} ("Laser Controls 2"), "Initialize"=TRUE) -> ()  [unwired: 12 in, 1 out]
      }
      frame "Start FPGA Acquisition" {
        n223 = Unbundle By Name(w414) -> ("Scan Type"=w413:enum16{"Sample Scanning", "Beam Scanning"})
        n224 = case shown="\"Beam Scanning\"" w413 {
          tunnel: w414 -> [w419 w426]
          tunnel: w412 -> [w418 w427]
          frame "Sample Scanning", Default {
            n225 = vi-ref "FPGA Sample Scanning V1.vi"() -> (w422:refnum<vi>)
            n226 = property class="VI Interface Type 0"(reference=w422) -> ("Path"=w420:path)  [unwired: 1 in, 2 out]
            n227 = Open VI Reference(type specifier VI Refnum (for type only)=w422, vi path=w420, options=128) -> (vi reference=w423:refnum<vi>)  [unwired: 3 in, 1 out]
            n228 = call-by-ref "Start Asynchronous Call"(reference=w423, "Detectors"=w418, "Image Acquisition Parameters"=w419) -> (reference out=w424:refnum<vi>)  [unwired: 2 in, 1 out]
            n229 = Close Reference(reference=w424) -> ()  [unwired: 1 in, 1 out]
          }
          frame "Beam Scanning" {
            n230 = vi-ref "FPGA Beam Scanning V1.vi"() -> (w425:refnum<vi>)
            n231 = property class="VI Interface Type 0"(reference=w425) -> ("Path"=w429:path)  [unwired: 1 in, 2 out]
            n232 = Open VI Reference(type specifier VI Refnum (for type only)=w425, vi path=w429, options=128) -> (vi reference=w428:refnum<vi>)  [unwired: 3 in, 1 out]
            n233 = call-by-ref "Start Asynchronous Call"(reference=w428, "Detectors"=w427, "Image Acquisition Parameters"=w426) -> (reference out=w431:refnum<vi>)  [unwired: 2 in, 1 out]
            n234 = Close Reference(reference=w431) -> ()  [unwired: 1 in, 1 out]
          }
        }
      }
    }
  }
  n235 = local write "Quit"(w3) -> ()
